vi "Test HTTP.vi"() -> ()   [LabVIEW 2016]
uses:
  <vilib>/addons/_JKI Toolkits/Caraya/classes/Test/Test.lvclass
panel:
  in  "error in":errorcluster
  out "error out":errorcluster
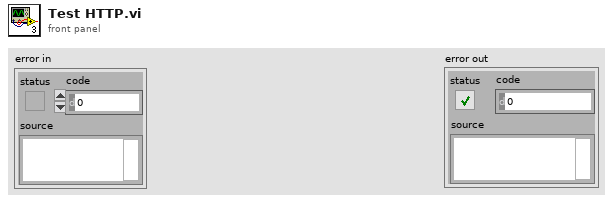
[diagram p1: front panel]
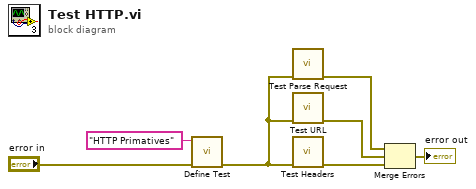
[diagram p0: block diagram]
diagram:
  n1 = call <vilib>:"Define Test.vi"("error in (no error)"="error in", "Label (VI Title)"="HTTP Primatives") -> ("error out"=w6:errorcluster)  [unwired: 9 in]
  n2 = call "Test Parse Request.vi"("error in (no error)"=w6) -> ("error out"=w5:errorcluster)  [unwired: 10 in]
  n3 = call "Test URL.vi"("error in (no error)"=w6) -> ("error out"=w4:errorcluster)  [unwired: 10 in]
  n4 = call "Test Headers.vi"("error in"=w6) -> ("error out"=w3:errorcluster)  [unwired: 10 in]
  n5 = Merge Errors(w5, w4, w3) -> (→"error out":errorcluster)
